vi "Calculate Viscocity.vi"(1 "Gas":T1(ring), 2 "T(K)":dbl=223.1) -> (0 "mu (Pa*s)":dbl=1.4685620043524856e-05)   [LabVIEW 2015, in "Atmospheric Library.lvlib"]
doc: "Calculate the viscosity of various gasses using the Sutherland formula. Viscosity is a function strictly of the temperature of the gas."
uses:
  Atmospheric Library.lvlib
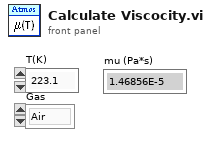
[diagram p1: front panel]
types:
  T1 = enum16{"Air", "N2", "O2", "CO2", "CO", "H2", "NH3", "SO2", "He"}
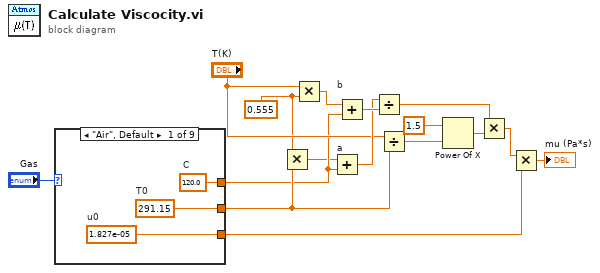
[diagram p0: block diagram]
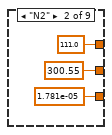
[diagram p2: hidden frame]
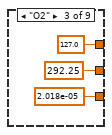
[diagram p3: hidden frame]
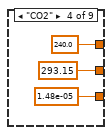
[diagram p4: hidden frame]
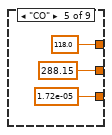
[diagram p5: hidden frame]
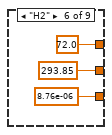
[diagram p6: hidden frame]
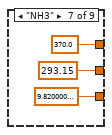
[diagram p7: hidden frame]
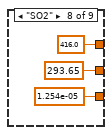
[diagram p8: hidden frame]
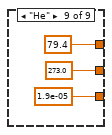
[diagram p9: hidden frame]
diagram:
  w3 = 0.555 ("y")
  n1 = case shown="\"Air\", Default" "Gas" {
    tunnel: [w19 111.0 127.0 240.0 118.0 72.0 370.0 416.0 79.4] -> w2
    tunnel: [w18 300.55 292.25 293.15 288.15 293.85 293.15 293.65 273.0] -> w4
    tunnel: [w17 1.781e-05 2.018e-05 1.48e-05 1.72e-05 8.76e-06 9.820000000000001e-06 1.254e-05 1.9e-05] -> w8
    frame "Air", Default {
      w17 = 1.827e-05  # u0
      w18 = 291.15  # T0
      w19 = 120.0  # C
    }
    frame "N2" {
    }
    frame "O2" {
    }
    frame "CO2" {
    }
    frame "CO" {
    }
    frame "H2" {
    }
    frame "NH3" {
    }
    frame "SO2" {
    }
    frame "He" {
    }
  }
  n2 = Multiply(x=w3, y=w4) -> (x*y=w1:dbl)
  n3 = Multiply(x="T(K)", y=w3) -> (x*y=w5:dbl)
  n4 = Add "a"(x=w1, y=w2) -> (x+y=w12:dbl)
  n5 = Add "b"(x=w5, y=w2) -> (x+y=w13:dbl)
  n6 = Divide(x=w12, y=w13) -> (x/y=w11:dbl)
  n7 = Divide(x="T(K)", y=w4) -> (x/y=w15:dbl)
  n8 = Power Of X(1:w15, 2:1.5 ("y")) -> (0:w10:dbl)
  n9 = Multiply(x=w11, y=w10) -> (x*y=w9:dbl)
  n10 = Multiply(x=w9, y=w8) -> (x*y=→"mu (Pa*s)":dbl)
